vi "Read.vi"(11 "VolatusNodeValue in":refnum<class "VolatusNodeValue.lvclass">) -> (2 "Node":refnum<class "Node.lvclass">)   [LabVIEW 2020, in "Volatus.lvlib" / "VolatusNodeValue.lvclass"]
uses:
  VolatusNodeValue.lvclass
  VolatusNodeValue.lvclass/VolatusNodeValue.ctl
  VolatusConfig/Node/Node.lvclass
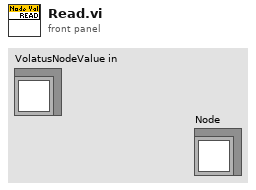
[diagram p1: front panel]
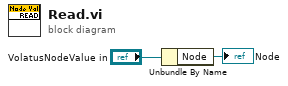
[diagram p0: block diagram]
diagram:
  n1 = Unbundle By Name("VolatusNodeValue in") -> ("Node"=→"Node":refnum<class "Node.lvclass">)
